vi "ProcessSensorData.vi"(8 "error in (no error)":errorcluster, 11 "PmuAnalysis":refnum<class "PmuDelay.lvclass">) -> (0 "error out":errorcluster, 2 "TimedOut":bool, 3 "PMUAnalysis":refnum<class "PmuDelay.lvclass">)   [LabVIEW 2018, in "AnalysisPlugins.lvlib" / "PmuDelay.lvclass"]
uses:
  PmuDelay.lvclass
  C:/projects/ICDAS/NistPluggableModules/Analysis/AnalysisPlugins/AnalysisPluginBaseClass/AnalysisPluginsBase.lvclass
  C:/projects/ICDAS/NistPluggableModules/Analysis/AnalysisPlugins/PmuAnalysisClass/PmuAnalysis.lvclass
  AnalysisPluginBaseClass/AnalysisPluginsBase.lvclass/AnalysisPluginsBase.ctl
  PmuAnalysisClass/Typedefs/PmuData.ctl
  PmuAnalysisClass/PmuAnalysis.lvclass/PmuAnalysis.ctl
  AnalysisPluginBaseClass/Accessors/Write AnalysisTime.vi
  PmuAnalysisClass/Accessors/Write PmuReport.vi
  AnalysisPluginBaseClass/Accessors/Read SensorQue.vi
  <vilib>/Utility/error.llb/Error Cluster From Error Code.vi
  <vilib>/ErrorRing/Error Ring.xnode
  PmuAnalysisClass/PmuAnalysis.lvclass
panel:
  out "Waveform Chart":dbl(graph)
  out "time stamp":timestamp format="%^<%.3X\n%x>T"
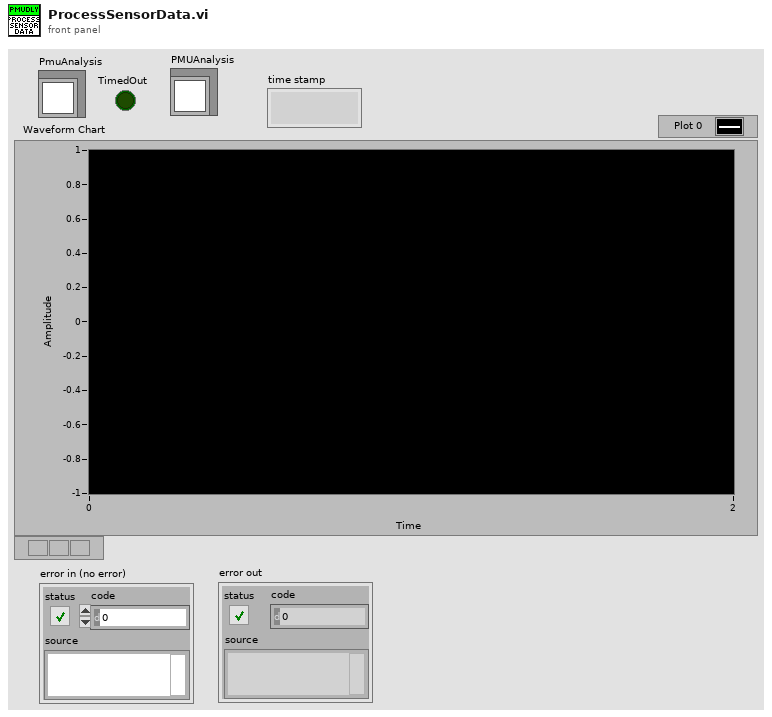
[diagram p1: front panel]
types:
  T1 = typedef "AnalysisPlugins.lvlib/PmuAnalysis.lvclass/PmuData.ctl" = cluster{"Timestamp":dbl, "Synx":cdb[], "Freq":dbl, "ROCOF":dbl, "ID":i16}
  T2 = typedef "SensorQueue.ctl" = refnum<queue>
  T3 = typedef "AnalysisPlugins.lvlib/AnalysisPluginsBase.lvclass/clSensorData.ctl" = cluster{"SensorType":string, "SensorData":variant, "TimeStamp":timestamp}
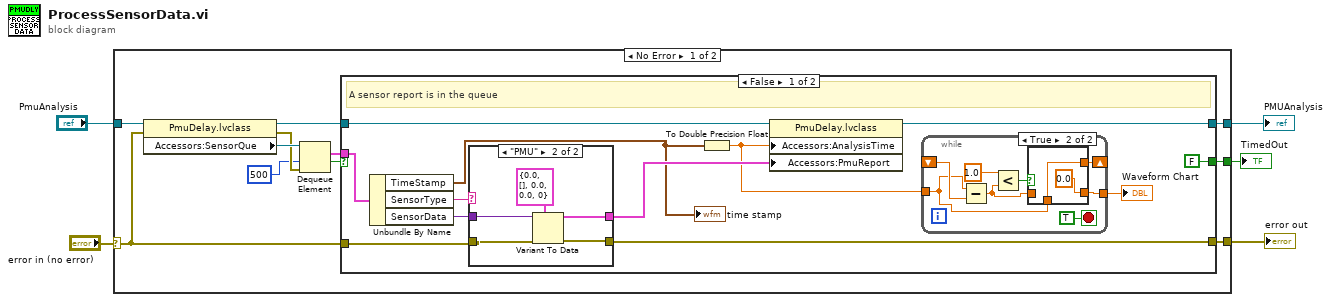
[diagram p0: block diagram]
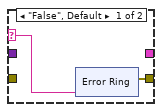
[diagram p3: hidden frame]
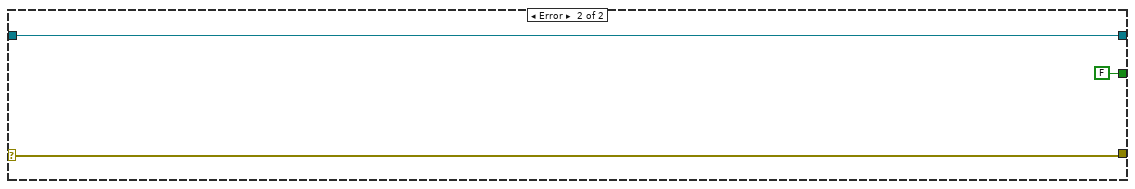
[diagram p5: hidden frame]
diagram:
  n1 = case shown="No Error" "error in (no error)" {
    selector: "error in (no error)" -> [w8 w59]
    tunnel: "PmuAnalysis" -> [w16 w60]
    tunnel: [w15 w60] -> w3
    tunnel: [w14 w59] -> w2
    tunnel: [w6 FALSE] -> w1
    frame No Error {
      n2 = property class="PmuDelay.lvclass"(reference=w16, error in=w8) -> (reference out=w13:refnum<class "PmuDelay.lvclass">, error out=w11:errorcluster, "Accessors:SensorQue"=w12:T2)
      n3 = Dequeue Element(queue=w12, timeout in ms (-1)=500, error in (no error)=w11) -> (element=w9:T3, timed out?=w7:bool)  [unwired: 2 out]
      n4 = case shown="False" w7 {
        selector: w7 -> [_ w55]
        tunnel: [w26 w57] -> w15
        tunnel: [w24 w56] -> w14
        tunnel: w13 -> [w23 w57]
        tunnel: w9 -> [w22 _]
        tunnel: w8 -> [w20 w56]
        tunnel: [FALSE w55] -> w6
        frame False {
          # "A sensor report is in the queue"
          n5 = Unbundle By Name(w22) -> ("TimeStamp"=w18:timestamp, "SensorType"=w28:string, "SensorData"=w27:variant)
          "time stamp" <- w18
          n6 = case shown="\"PMU\"" w28 {
            selector: w28 -> [w41 _]
            tunnel: [w42 w51] -> w24
            tunnel: w27 -> [_ w54]
            tunnel: w20 -> [_ w53]
            tunnel: [_ w50] -> w25
            frame "False", Default {
              n7 = xnode "Error Ring"("parameter 0"=w41) -> ("error out"=w42:errorcluster)
            }
            frame "PMU" {
              n8 = Variant To Data(error in=w53, type=T1 {"Timestamp"=0.0, "Synx"=[], "Freq"=0.0, "ROCOF"=0.0, "ID"=0} ("PmuReport"), Variant=w54) -> (data=w50:T1, error out=w51:errorcluster)
            }
          }
          n9 = To Double Precision Float(number=w18) -> (double precision float=w17:dbl)
          n10 = property class="PmuDelay.lvclass"(reference=w23, "Accessors:AnalysisTime"=w17, "Accessors:PmuReport"=w25) -> (reference out=w26:refnum<class "PmuDelay.lvclass">)  [unwired: 1 in, 1 out]
          n11 = while {
            tunnel: w17 -> [w30]
            shift-right: [w29] -> _
            shift-left: _ -> [w32]
            tunnel: [w31] -> w21
            stop <- TRUE stop-if-true
            n12 = Subtract(x=w30, y=w32) -> (x-y=w33:dbl)
            n13 = Less?(x=1.0, y=w33) -> (x < y?=w34:bool)
            n14 = case shown="True" w34 {
              tunnel: w33 -> [w38 _]
              tunnel: [w38 0.0] -> w31
              tunnel: w30 -> [w37 w39]
              tunnel: [w37 w39] -> w29
              frame False {
              }
              frame True {
              }
            }
          }
          "Waveform Chart" <- w21
        }
        frame True {
          # "Queue Timed out, allow the loop to run to check for stop state"
        }
      }
    }
    frame Error {
    }
  }
  "PMUAnalysis" <- w3
  "error out" <- w2
  "TimedOut" <- w1
